vi "runServer.vi"(8 "error in (no error)":errorcluster, 11 "TcpServerTel in":refnum<class "TcpServerTel.lvclass">) -> (0 "error out (no error)":errorcluster, 3 "TcpServerTel out":refnum<class "TcpServerTel.lvclass">)   [LabVIEW 2018, in "TcpServerTel.lvclass"]
doc: "Run the TCP Server Telemetry.\n\nNOTE: Server Queue and Client Queue are destroyed in \"stop server\" state inside of tcpServerStateMachine.vi"
uses:
  TcpServerTel.lvclass
  home/pcortes/github/ts_labview_tcp_json/src/TcpServerBase/TcpServerBase.lvclass
  TcpServerBase/TcpServerBase.lvclass/TcpServerBase.ctl
  TcpServerBase/TcpServerBase.lvclass
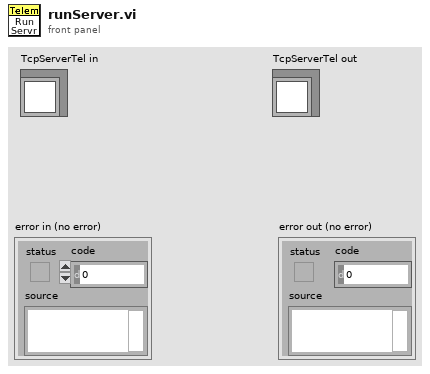
[diagram p1: front panel]
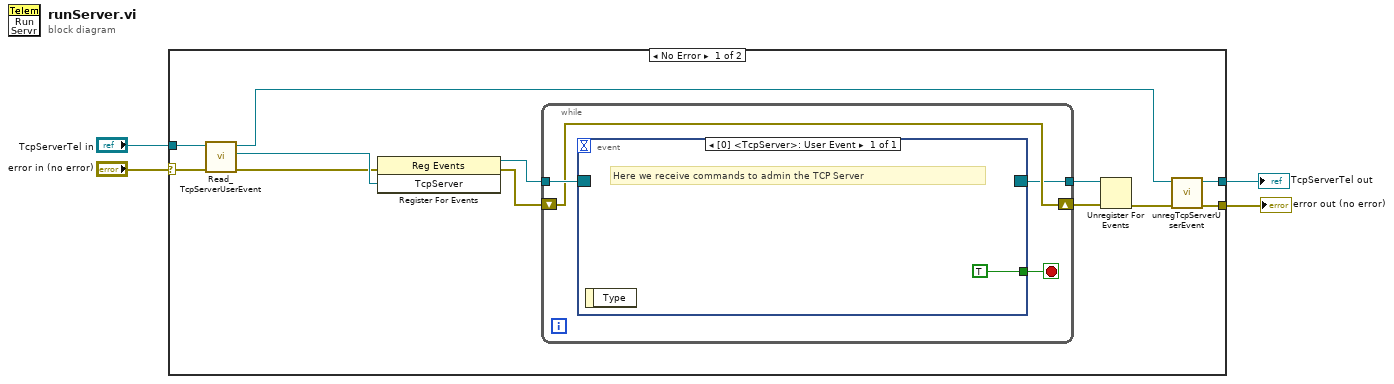
[diagram p0: block diagram]
diagram:
  n1 = case shown="No Error" "error in (no error)" {
    selector: "error in (no error)" -> [w10 w23]
    tunnel: [w8 w22] -> w3
    tunnel: [w7 w23] -> w2
    tunnel: "TcpServerTel in" -> [w5 w22]
    frame No Error {
      n2 = call "Read_TcpServerUserEvent.vi"("error in (no error)"=w10, "TcpServerBase in"=w5) -> ("error out"=w15:errorcluster, "TcpServer"=w16:refnum<user-event>, "TcpServerBase out"=w9:refnum<class "TcpServerTel.lvclass">)  [unwired: 7 in]
      n3 = register-events(error in=w15, w16) -> (reference out=w14:refnum<event-registration>, error out=w13:errorcluster)  [unwired: 1 in]
      n4 = while {
        tunnel: w14 -> [w20]
        shift-right: [w18] -> w12
        shift-left: w13 -> [w18]
        tunnel: [w17] -> w11
        stop <- w19 stop-if-true
        n5 = event shown="[0] <TcpServer>: User Event" {
          selector: w20 -> [_]
          dyn-events: [_] -> w17
          timeout: _ -> [_]
          tunnel: [TRUE] -> w19
          event User Event {
            # "Here we receive commands to admin the TCP Server"
            n6 = event-data() -> ()  [unwired: 1 in, 1 out]
          }
        }
      }
      n7 = Unregister For Events(event registration refnum=w11, error in=w12) -> (error out=w6:errorcluster)
      n8 = call "unregTcpServerUserEvent.vi"("error in (no error)"=w6, "tcpServerBase in"=w9) -> ("error out"=w7:errorcluster, "tcpServerBase out"=w8:refnum<class "TcpServerTel.lvclass">)  [unwired: 8 in]
    }
    frame Error {
    }
  }
  "error out (no error)" <- w2
  "TcpServerTel out" <- w3
